vi "Calculate Motion Profile Length.vi"(8 "error in (no error)":errorcluster, 11 "Motion Profile Generator in":refnum<class "Motion Profile Generator.lvclass">) -> (0 "error out":errorcluster, 1 "Duration (s)":dbl, 2 "Steps":i32, 3 "Motion Profile Generator out":refnum<class "Motion Profile Generator.lvclass">, 4 "Time Between Points (ms)":dbl)   [LabVIEW 2019, in "Motion Profile Generator.lvclass"]
uses:
  Motion Profile Generator.lvclass
  Motion Profile Generator.lvclass/Motion Profile Generator.ctl
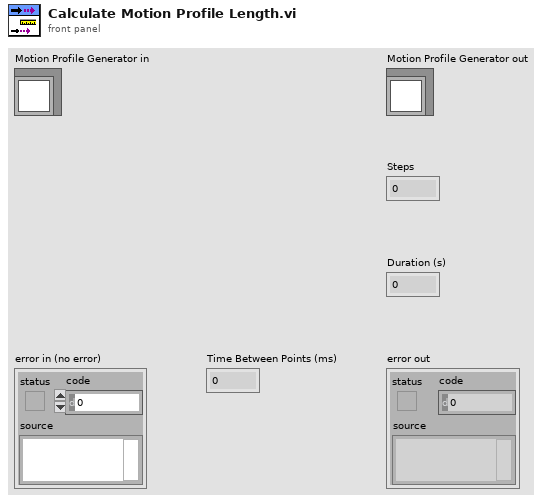
[diagram p1: front panel]
types:
  T1 = typedef "Motion Profile Generator.lvclass/Motion Profile Point.ctl" = cluster{"Position (in)":dbl, "Velocity (in/s)":dbl, "Duration (ms)":dbl}
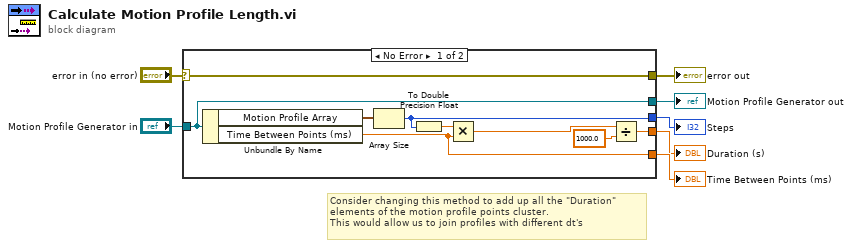
[diagram p0: block diagram]
diagram:
  # "Consider changing this method to add up all the \"Duration\"\nelements of the motion profile points cluster.\nThis would allow us to join profiles with different dt's"
  n1 = case shown="No Error" "error in (no error)" {
    selector: "error in (no error)" -> [w16 w18]
    tunnel: [w16 w18] -> w6
    tunnel: [w15 w17] -> w4
    tunnel: "Motion Profile Generator in" -> [w15 w17]
    tunnel: [w13 _] -> w3
    tunnel: [w11 _] -> w2
    tunnel: [w9 _] -> w1
    frame No Error {
      n2 = Unbundle By Name(w15) -> ("Motion Profile Array"=w14:T1[], "Time Between Points (ms)"=w13:dbl)
      n3 = Array Size(array=w14) -> (size(s)=w11:i32)
      n4 = To Double Precision Float(number=w11) -> (double precision float=w10:dbl)
      n5 = Multiply(x=w10, y=w13) -> (x*y=w12:dbl)
      n6 = Divide(x=w12, y=1000.0) -> (x/y=w9:dbl)
    }
    frame Error {
    }
  }
  "error out" <- w6
  "Motion Profile Generator out" <- w4
  "Duration (s)" <- w1
  "Steps" <- w2
  "Time Between Points (ms)" <- w3
